vi "Keithley2100.destructor.vi"(0 "i ref in":refnum<vi>, 5 "error in (no error)":errorcluster) -> (19 "error out":errorcluster)   [LabVIEW 2014, in "Keithley2100.lvlib"]
doc: "This is the destructor of a class.\n\nLicense Agreement for this software:\n\nCopyright (C)\nGesellschaft für Schwerionenforschung, GSI\nPlanckstr. 1\n64291 Darmstadt\nGermany\n\nContact: D.Beck@gsi.de \n\nThis program is free software; you can redistribute it and/or modify it under the terms of the \nGNU General Public License as published by the Free Software Foundation; either version 2 of \nthe license, or (at your option) any later version.\n\nThis program is distributed in the hope that it will be useful, but WITHOUT ANY WARRANTY; \nwithout even the implied warranty of MERCHANTABILITY or FITNESS FOR A PARTICULAR PURPOSE. See the GNU General License for more details (http://www.gnu.org).\n\nGesellschaft für Schwerionenforschung, GSI\nPlanckstr. 1, 64291 Darmstadt, Germany\nFor all questions and ideas contact: M.Richter@gsi.de, H.Brand@gsi.de or D.Beck@gsi.de.\nLast update: 16-JUN-2004"
uses:
  Keithley2100.lvlib
  CS_Core/CSApplicationBaseClasses/DeviceBase/DeviceBase.lvlib
  CSlibraries-extern/DimLVEvent/LVDimInterface/LVDimInterface.lvlib
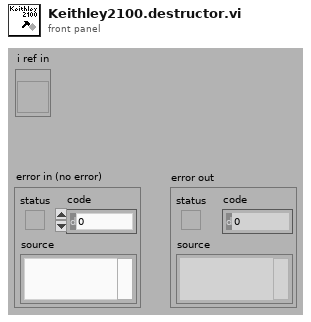
[diagram p1: front panel]
types:
  T1 = typedef "Keithley2100.lvlib/Keithley2100.i attribute.ctl" = cluster{"Custom Range":dbl, "Threshold Range":dbl, "VISA resource name":refnum<visa-resource-name>, "Auto Range":bool, "Digital Filter Readings":i32, "Digital Filter":u16, "NPLC":u16, "Display on":u16, "Resolution":u16, "Beaper enabled":bool, "MeasurementID":i32}
  T2 = enum16{"SetAttribute", "GetAttribute", "CreateAttribute", "DestroyAttribute", "DestroyAllAtributes"}
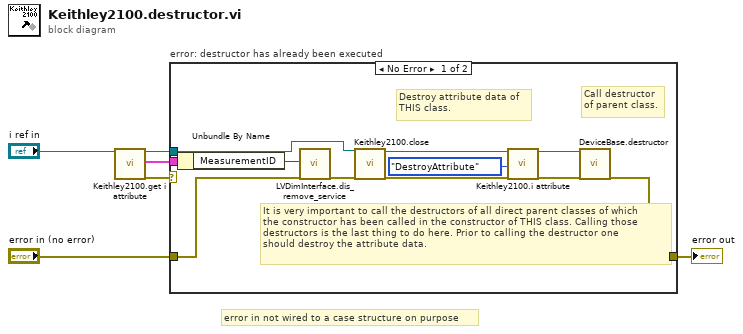
[diagram p0: block diagram]
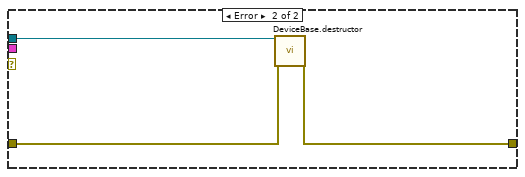
[diagram p2: hidden frame]
diagram:
  # "error in not wired to a case structure on purpose"
  n1 = call "Keithley2100.get i attribute.vi"("i ref in"="i ref in") -> ("i ref out"=w2:refnum<vi>, "i attribute"=w1:T1, "error out"=w3:errorcluster)  [unwired: 16 in]
  n2 = case "error: destructor has already been executed" shown="No Error" w3 {
    tunnel: [w14 w18] -> w6
    tunnel: "error in (no error)" -> [w9 w19]
    tunnel: w2 -> [w7 w20]
    tunnel: w1 -> [w11 _]
    frame No Error {
      # "It is very important to call the destructors of all direct parent classes of which\nthe constructor has been called in the constructor of THIS class. Calling those\ndestructors is the last thing to do here. Prior to calling the destructor one \nshould destroy the attribute data."
      # "Destroy attribute data of \nTHIS class."
      # "Call destructor\nof parent class."
      n3 = Unbundle By Name(w11) -> ("MeasurementID"=w10:i32)
      n4 = call "LVDimInterface.dis_remove_service.vi"("my_serviceID"=w10, "error in (no error)"=w9) -> ("error out"=w8:errorcluster)  [unwired: 17 in]
      n5 = call "Keithley2100.close.vi"("i ref in"=w7, "error in (no error)"=w8) -> ("i refout"=w13:refnum<vi>, "error out"=w12:errorcluster)  [unwired: 16 in]
      n6 = call "Keithley2100.i attribute.vi"("VI Refnum"=w13, "Action"=T2."DestroyAttribute", "error in (no error)"=w12) -> ("VI Refnum out"=w16:refnum<vi>, "error out"=w15:errorcluster)  [unwired: 14 in, 1 out]
      n7 = call "DeviceBase.destructor.vi"("i ref in"=w16, "error in (no error)"=w15) -> ("error out"=w14:errorcluster)  [unwired: 17 in]
    }
    frame Error {
      n8 = call "DeviceBase.destructor.vi"("i ref in"=w20, "error in (no error)"=w19) -> ("error out"=w18:errorcluster)  [unwired: 17 in]
    }
  }
  "error out" <- w6
